vi "save_data_queue.vi"() -> ()   [LabVIEW 2024]
panel:
  out "Waveform Chart 2":cluster{"N1":dbl, "N2":dbl}(graph)
  out "Waveform Chart":cluster{"N1":dbl, "N2":dbl}(graph)
  out "# elements in queue":i32
  in  "ms Consumidor":u32=200
  in  "ms Generador":u32=100
  in  "stop":bool
  in  "Cluster":cluster{"N1":dbl, "N2":dbl}
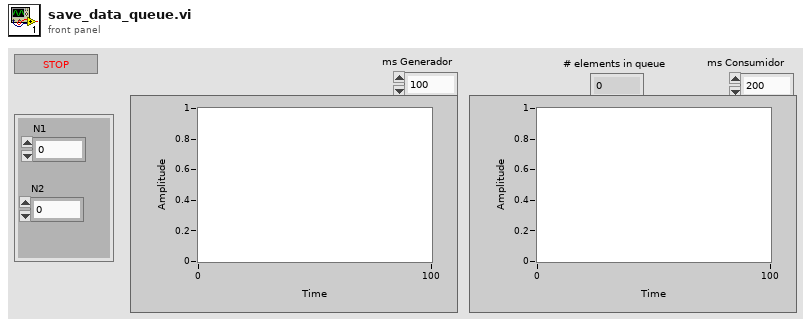
[diagram p1: front panel]
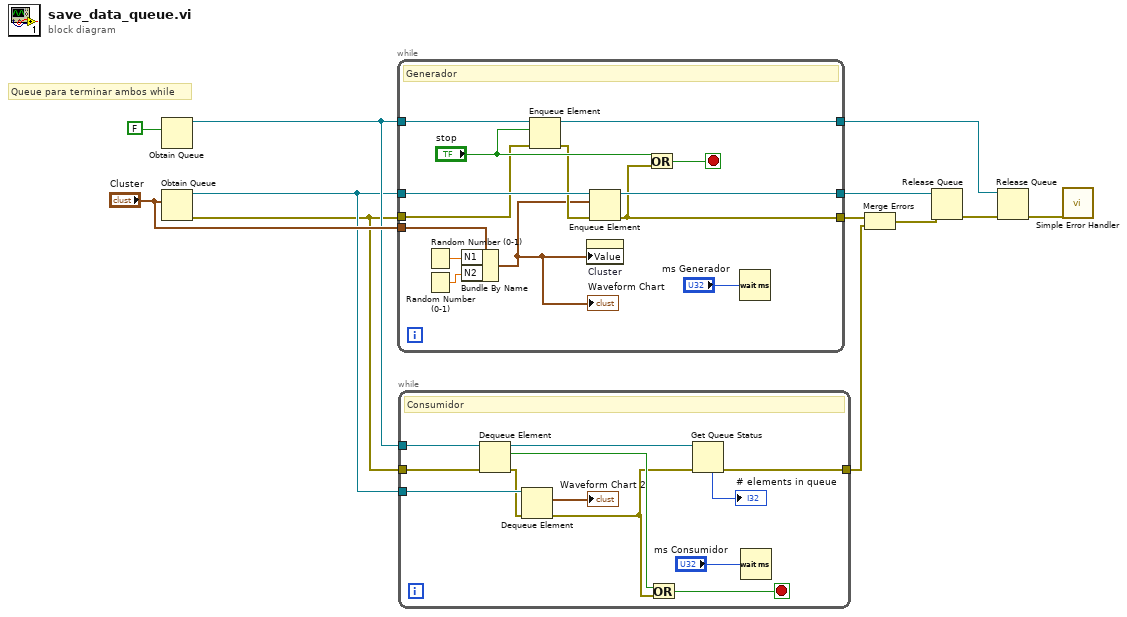
[diagram p0: block diagram]
diagram:
  # "Queue para terminar ambos while"
  n1 = Obtain Queue(element data type=FALSE) -> (queue out=w8:refnum<queue>)  [unwired: 4 in, 2 out]
  n2 = Obtain Queue(element data type="Cluster") -> (queue out=w7:refnum<queue>, error out=w6:errorcluster)  [unwired: 4 in, 1 out]
  n3 = while {
    tunnel: w8 -> [w25]
    tunnel: w7 -> [w24]
    tunnel: "Cluster" -> [w23]
    tunnel: [w20] -> w9
    tunnel: [w19] -> w10
    tunnel: w6 -> [w16]
    tunnel: [w15] -> w5
    stop <- w18 stop-if-true
    # "Generador"
    n4 = Random Number (0-1)() -> (number: 0 to 1=w14:dbl)
    n5 = Random Number (0-1)() -> (number: 0 to 1=w22:dbl)
    n6 = Bundle By Name(cluster=w23, "N1"=w14, "N2"=w22) -> (w13:cluster{"N1":dbl, "N2":dbl})
    "Waveform Chart" <- w13
    n7 = Enqueue Element(queue=w25, element="stop", error in (no error)=w16) -> (queue out=w20:refnum<queue>, error out=w17:errorcluster)  [unwired: 1 in, 1 out]
    n8 = property on="Cluster" class="Clust (strict)"("Value"=w13) -> ()  [unwired: 2 in, 2 out]
    n9 = Enqueue Element(queue=w24, element=w13, error in (no error)=w17) -> (queue out=w19:refnum<queue>, error out=w15:errorcluster)  [unwired: 1 in, 1 out]
    n10 = Or(x="stop", y=w15) -> (x .or. y?=w18:bool)
    n11 = Wait (ms)(milliseconds to wait="ms Generador") -> ()  [unwired: 1 out]
  }
  n12 = while {
    tunnel: w8 -> [w37]
    tunnel: w7 -> [w36]
    tunnel: w6 -> [w32]
    tunnel: [w27] -> w1
    stop <- w35 stop-if-true
    # "Consumidor"
    n13 = Dequeue Element(queue=w37, error in (no error)=w32) -> (queue out=w30:refnum<queue>, element=w34:bool, error out=w33:errorcluster)  [unwired: 1 in, 1 out]
    n14 = Dequeue Element(queue=w36, error in (no error)=w33) -> (element=→"Waveform Chart 2":cluster{"N1":dbl, "N2":dbl}, error out=w28:errorcluster)  [unwired: 1 in, 2 out]
    n15 = Or(x=w34, y=w28) -> (x .or. y?=w35:bool)
    n16 = Get Queue Status(queue=w30, error in (no error)=w28) -> (error out=w27:errorcluster, # elements in queue=→"# elements in queue":i32)  [unwired: 1 in, 6 out]
    n17 = Wait (ms)(milliseconds to wait="ms Consumidor") -> ()  [unwired: 1 out]
  }
  n18 = Merge Errors(w5, w1) -> (w2:errorcluster)
  n19 = Release Queue(queue=w10, error in (no error)=w2) -> (error out=w4:errorcluster)  [unwired: 1 in, 2 out]
  n20 = Release Queue(queue=w9, error in (no error)=w4) -> (error out=w3:errorcluster)  [unwired: 1 in, 2 out]
  n21 = call <vilib>:"Simple Error Handler.vi"("error in (no error)"=w3) -> ()  [unwired: 4 in, 5 out]
